vi "texture_test_packedu8.vi"() -> ()   [LabVIEW 2010]
uses:
  <vilib>/picture/picture.llb/Draw True-Color Pixmap.vi
panel:
  out "preview":picture
  out "packet sent to hologram engine":string
  in  "Texture to send":u32[][](array[colorbox])
  # "This demo shows the hologram engine being used to render a bitmap to the screen.  We have used a similar program to perform \"ghost imaging\" experiments.  The advantage of using OpenGL is that we can synchronise with the monitor refresh rate to achieve high speed display."
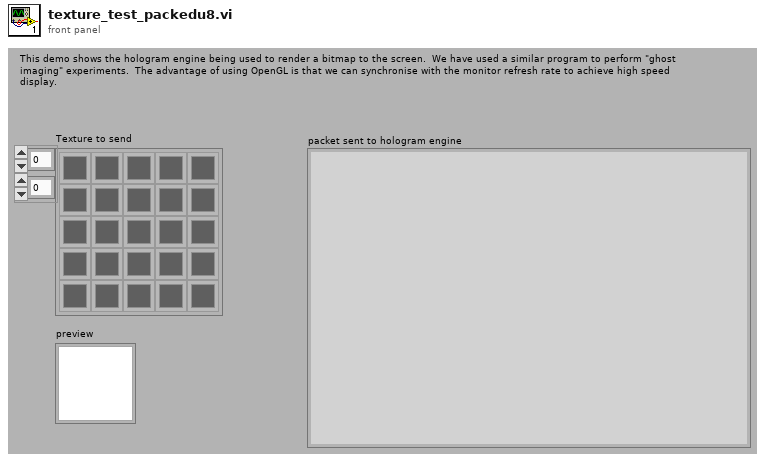
[diagram p1: front panel]
types:
  T1 = enum16{"big-endian, network order", "native, host order", "little-endian"}
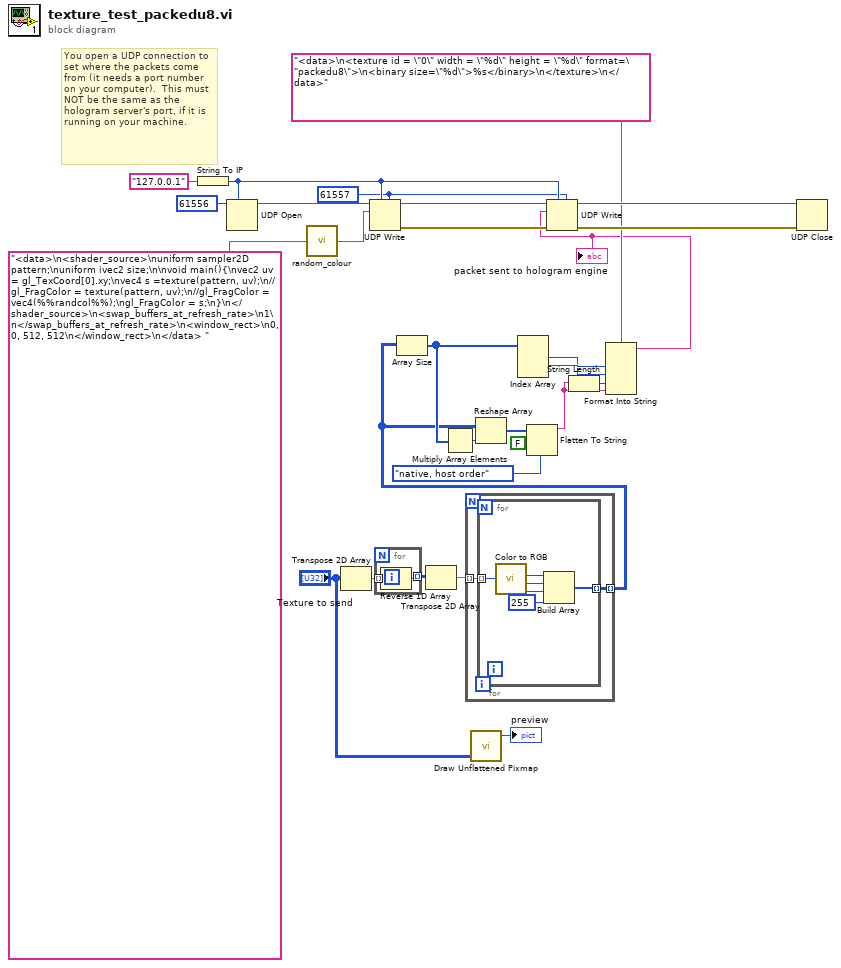
[diagram p0: block diagram]
diagram:
  w18 = u16 61557 ("port")
  # "You open a UDP connection to set where the packets come from (it needs a port number on your computer).  This must NOT be the same as the hologram server's port, if it is running on your machine."
  n1 = String To IP(1:"127.0.0.1" ("name")) -> (0:w19:u32)
  n2 = UDP Open(7:w19, 11:u16 61556 ("port")) -> (port=w28:refnum<k16>)  [unwired: 3 in, 2 out]
  n3 = call "random_colour.vi"("string in"="<data>\n<shader_source>\nuniform sampler2D pattern;\nuniform ivec2 size;\n\nvoid main(){\nvec2 uv = gl_TexCoord[0].xy;\nvec4 s =texture(pattern, uv);\n//gl_FragColor = texture(pattern, uv);\n//gl_FragColor = vec4(%%randcol%%);\ngl_FragColor = s;\n}\n</shader_source>\n<swap_buffers_at_refresh_rate>\n1\n</swap_buffers_at_refresh_rate>\n<window_rect>\n0, 0, 512, 512\n</window_rect>\n</data> " ("data in")) -> ("string out, with %%randcol%% replaced with a 4-element colour"=w25:string)
  n4 = Transpose 2D Array(2D array="Texture to send") -> (transposed array=w6:u32[][])
  n5 = UDP Write(address=w19, port or service name=w18, connection ID=w28, data in=w25) -> (error out=w20:errorcluster, 3:w23:refnum<k16>)  [unwired: 2 in]
  n6 = for {
    tunnel: w6 -> [w30] mode=indexing
    tunnel: [w29] -> w5 mode=indexing
    n7 = Reverse 1D Array(array=w30) -> (reversed array=w29:u32[])
  }
  n8 = Transpose 2D Array(2D array=w5) -> (transposed array=w3:u32[][])
  n9 = for {
    tunnel: w3 -> [w31] mode=indexing
    tunnel: [w32] -> w4 mode=indexing
    n10 = for {
      tunnel: w31 -> [w38] mode=indexing
      tunnel: [w33] -> w32 mode=indexing
      n11 = call <vilib>:"Color to RGB.vi"("Color"=w38) -> ("R"=w35:u8, "G"=w37:u8, "B"=w36:u8)  [unwired: 1 out]
      n12 = Build Array(w35, w37, w36, u8 255 ("element")) -> (w33:u8[])
    }
  }
  n13 = Array Size(array=w4) -> (size(s)=w15:i32[])
  n14 = Multiply Array Elements(1:w15) -> (0:w16:i32)
  n15 = call-poly <vilib>:"Draw Unflattened Pixmap.vi"("data (RGB format)"="Texture to send") -> ("new picture"=→"preview":picture)  [unwired: 8 in]
  n16 = Reshape Array(w4, w16) -> (w9:u8[])
  n17 = Index Array(array=w15) -> (element #1=w12:i32, element #2=w13:i32)  [unwired: 3 in, 1 out]
  n18 = Flatten To String(anything=w9, prepend array or string size? (T)=FALSE, byte order (0:big-endian, network order)=T1."native, host order") -> (data string=w7:string)  [unwired: 1 in, 2 out]
  n19 = String Length(string=w7) -> (length=w8:i32)
  n20 = Format Into String(format string="<data>\n<texture id = \"0\" width = \"%d\" height = \"%d\" format=\"packedu8\">\n<binary size=\"%d\">%s</binary>\n</texture>\n</data>", w13, w12, w8, w7) -> (resulting string=w14:string)  [unwired: 2 in, 1 out]
  "packet sent to hologram engine" <- w14
  n21 = UDP Write(address=w19, port or service name=w18, connection ID=w23, data in=w14, 8:w20) -> (error out=w21:errorcluster, 3:w22:refnum<k16>)  [unwired: 1 in]
  n22 = UDP Close(connection ID=w22, 8:w21) -> ()  [unwired: 2 out]
